vi "Global DT per visualizzazione.vi"() -> ()   [LabVIEW 2019]
panel:
  in  "Dt resistomat":dbl[](array[numeric])
  in  "Dt resmeter":dbl[](array[numeric])
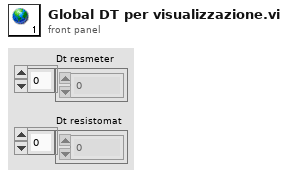
[diagram p1: front panel]
diagram:
